vi "Populate Tree.vi"(8 "error in":errorcluster, 10 "cDAQ Configs":T1[](array[typedef]), 11 "FP Controls":refnum<class "FP Controls.lvclass">) -> (0 "error out":errorcluster, 3 "FP Controls":refnum<class "FP Controls.lvclass">)   [LabVIEW 2012, in "Configuration Grandmaster.lvlib" / "FP Controls.lvclass"]
uses:
  FP Controls.lvclass
  Custom Ctrls/Master Cfg/ge_Cfg wChassis.ctl
  Class Chassis BOM/Chassis BOM.lvclass
  Class Chassis Cfg/ChassisCfg.lvclass
  Data Acquisition/Class Chassis Tasks/Chassis Tasks.lvclass
  SubVIs Main/Tree Control/Custom Ctrls/ge_ChassisTree.ctl
  FP Controls.lvclass/FP Controls.ctl
  Class Chassis BOM/Chassis BOM.lvclass/Chassis BOM.ctl
  Class Chassis BOM/Read Chassis Alias.vi
  Class Chassis BOM/Read HW Mods.vi
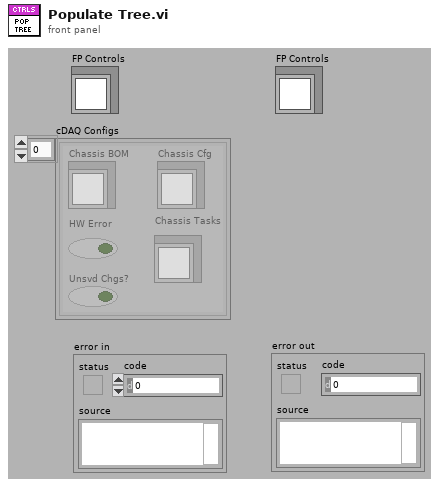
[diagram p1: front panel]
types:
  T1 = typedef "ge_Cfg wChassis.ctl" = cluster{"Chassis BOM":refnum<class "Chassis BOM.lvclass">, "Chassis Cfg":refnum<class "ChassisCfg.lvclass">, "Chassis Tasks":refnum<class "Chassis Tasks.lvclass">, "HW Error":bool, "Unsvd Chgs?":bool}
  T2 = typedef "ge_ChassisTree.ctl" = enum16{"Init", "Add Chassis", "Add Mod", "Close"}
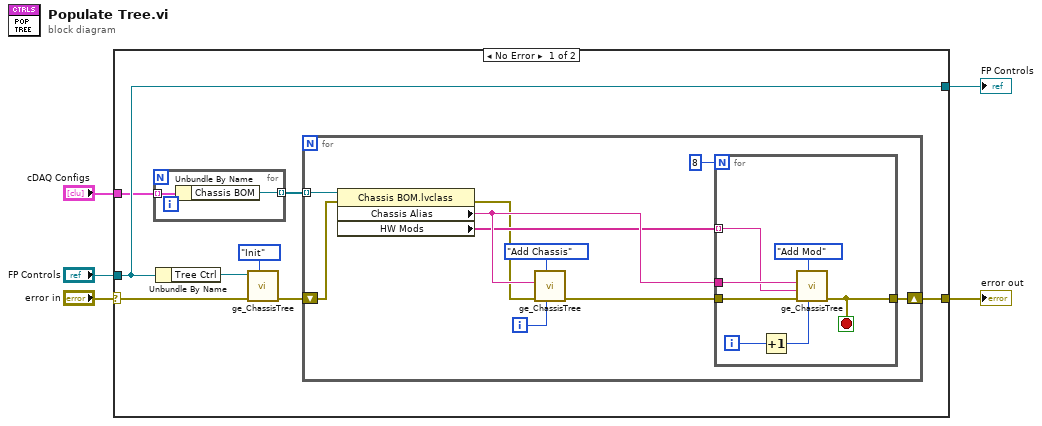
[diagram p0: block diagram]
diagram:
  n1 = case shown="No Error" "error in" {
    selector: "error in" -> [w9 w33]
    tunnel: "cDAQ Configs" -> [w7 _]
    tunnel: [w11 w33] -> w4
    tunnel: "FP Controls" -> [w8 w34]
    tunnel: [w8 w34] -> w1
    frame No Error {
      n2 = for {
        tunnel: w7 -> [w15] mode=indexing
        tunnel: [w14] -> w6 mode=indexing
        n3 = Unbundle By Name(w15) -> ("Chassis BOM"=w14:refnum<class "Chassis BOM.lvclass">)
      }
      n4 = Unbundle By Name(w8) -> ("Tree Ctrl"=w10:refnum<vi>)
      n5 = call "ge_ChassisTree.vi"("ge_TreeCmnd"=ge_ChassisTree."Init", "error in"=w9, "Hardware"=w10) -> ("error out"=w13:errorcluster)  [unwired: 8 in]
      n6 = for {
        shift-right: [w25] -> w11
        shift-left: w13 -> [w19]
        tunnel: w6 -> [w20] mode=indexing
        i -> [w21]
        n7 = property class="Chassis BOM.lvclass"(reference=w20, error in=w19) -> (error out=w16:errorcluster, "Chassis Alias"=w18:string, "HW Mods"=w17:string[])  [unwired: 1 out]
        n8 = call "ge_ChassisTree.vi"("Child Position"=w21, "ge_TreeCmnd"=ge_ChassisTree."Add Chassis", "error in"=w16, "Chassis Name"=w18) -> ("error out"=w24:errorcluster)  [unwired: 7 in]
        n9 = for {
          N: 8 -> [_]
          tunnel: w18 -> [w31]
          tunnel: [w28] -> w25
          tunnel: w24 -> [w29]
          tunnel: w17 -> [w26] mode=indexing
          i -> [w30]
          stop <- w28 stop-if-true
          n10 = Increment(x=w30) -> (x+1=w27:i32)
          n11 = call "ge_ChassisTree.vi"("Child Position"=w27, "ge_TreeCmnd"=ge_ChassisTree."Add Mod", "error in"=w29, "Module Name"=w26, "Chassis Name"=w31) -> ("error out"=w28:errorcluster)  [unwired: 6 in]
        }
      }
    }
    frame Error {
    }
  }
  "error out" <- w4
  "FP Controls" <- w1
